vi "GUI_FINAL.vi"() -> ()   [LabVIEW 2013]
uses:
  <vilib>/userdefined/High Color/IMAQdx.ctl
  <vilib>/Instr/_visa.llb/VISA Configure Serial Port (Instr).vi
  <vilib>/vision/driver/NI_Vision_Acquisition_Software.lvlib
panel:
  out "Temperatura Alta":bool
  out "Nivel Bajo":bool
  in  "CAMARA RETRO":bool
  out "luces":u8
  out "Gasolina":u8(slide) scale=0.0..100.0
  out "Capturaretro":T1(plugin-control)
  out "Direccional  Izquierda 2":bool
  out "Direccional Derecha 2":bool
  out "FRENO":bool
  out "LUZ DELANTERA":bool
  in  "ENCENDER":bool[](array[boolean])
  in  "VISA resource name":refnum<visa-resource-name>
  in  "stop":bool
  out "Hora":string
  out "Fecha":string
  out "velocidad":u8
  out "Km recorridos":u8
  out "nivel":u8
  out "temperatura":u8
  out "Vel":dbl(knob) scale=0.0..160.0
  out "Temperatura":dbl(knob) scale=0.0..100.0
  out "error out":errorcluster
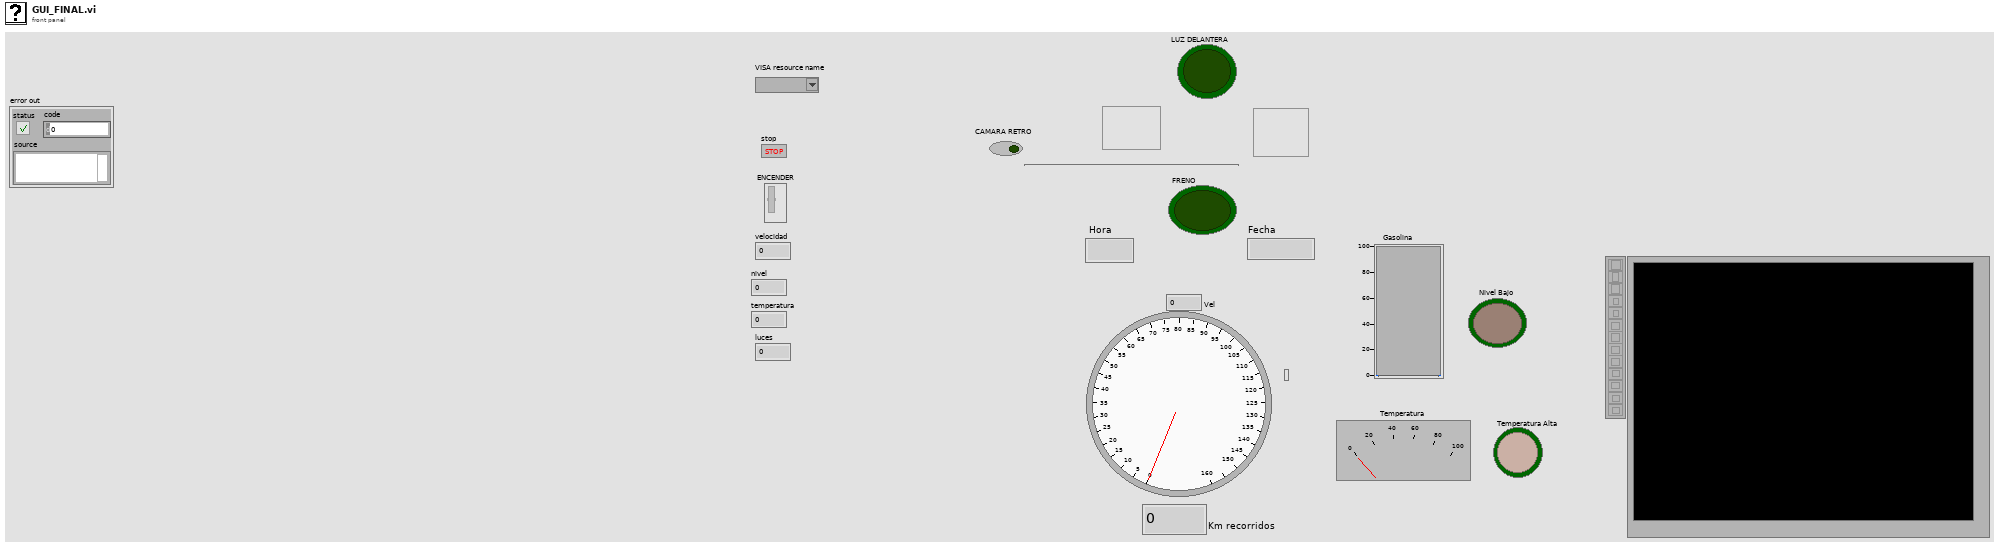
[diagram p1: front panel]
types:
  T1 = typedef "IMAQ Image.ctl" = refnum<image>
  T2 = typedef "IMAQdx.ctl" = refnum<k21>
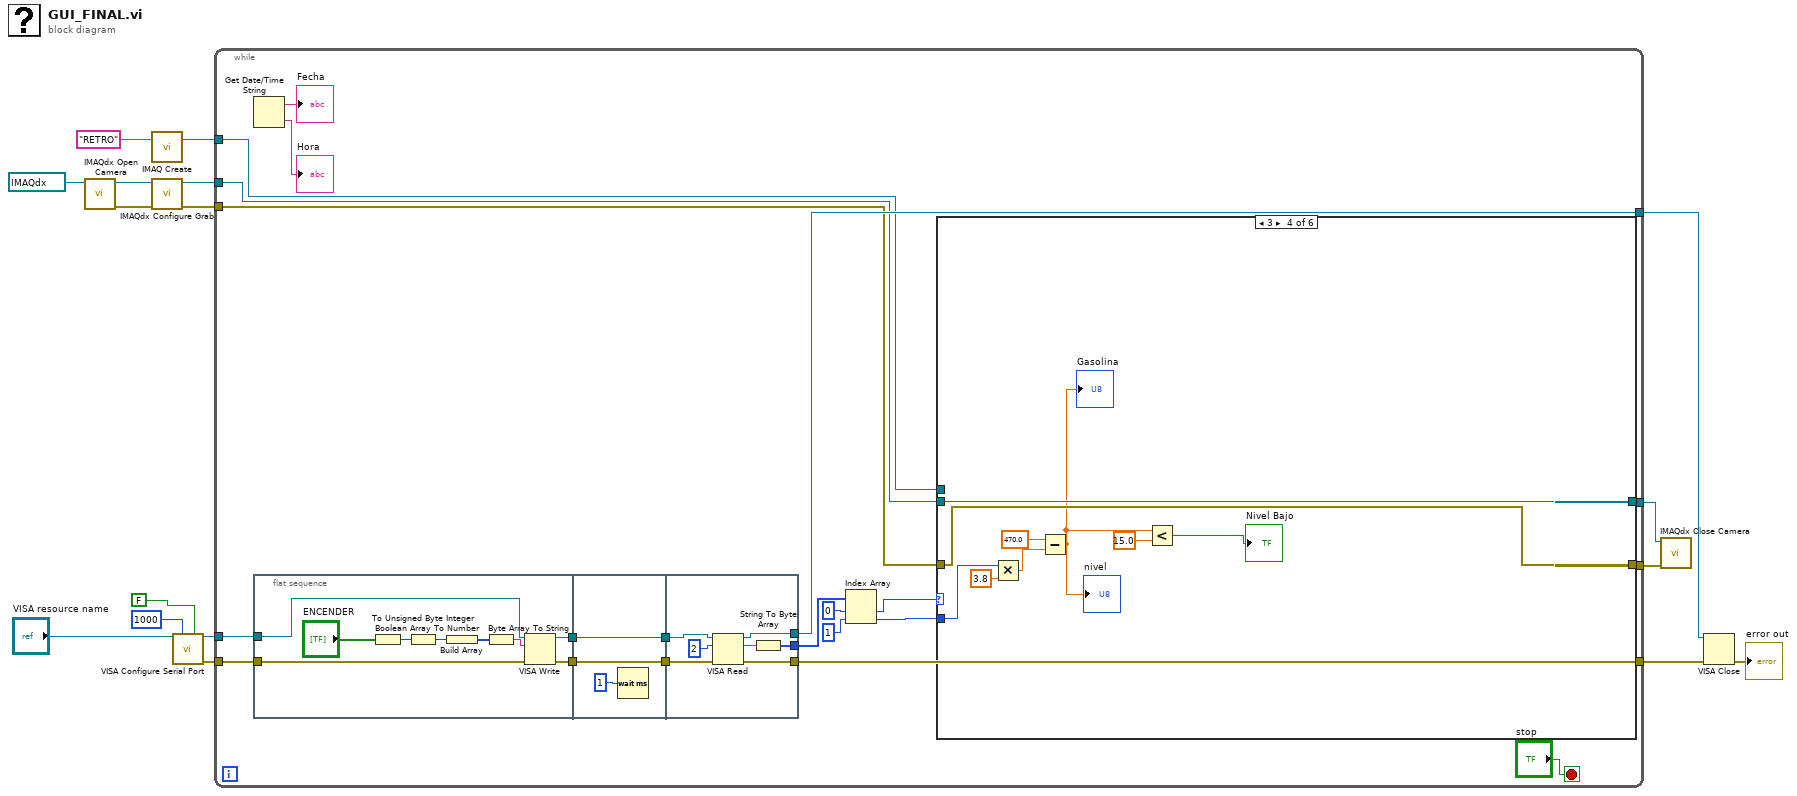
[diagram p0: block diagram]
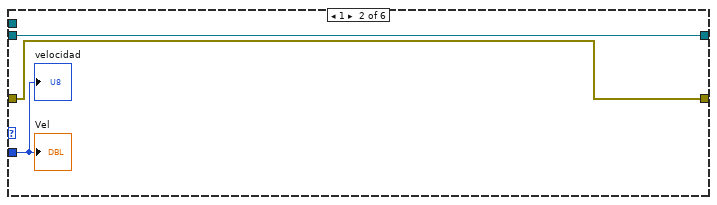
[diagram p3: hidden frame]
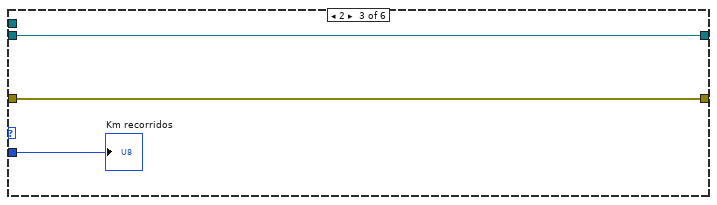
[diagram p4: hidden frame]
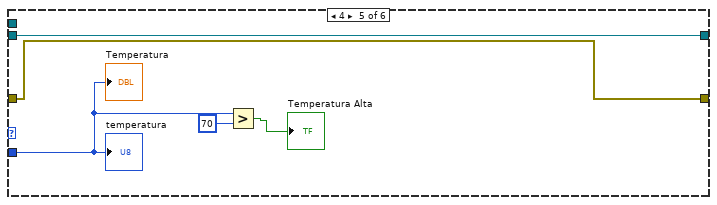
[diagram p5: hidden frame]
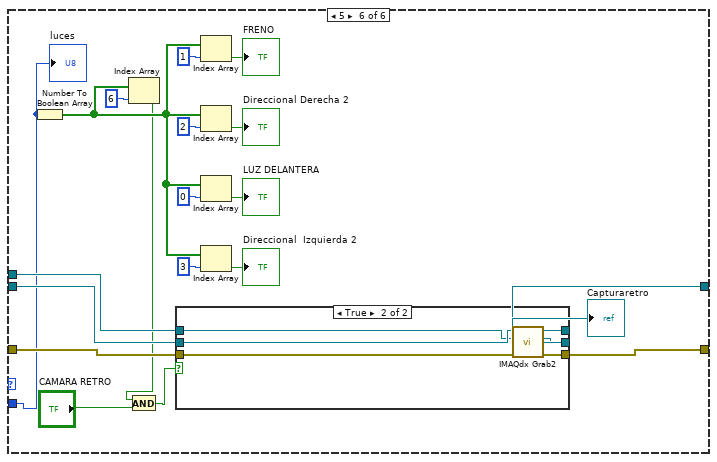
[diagram p6: hidden frame]
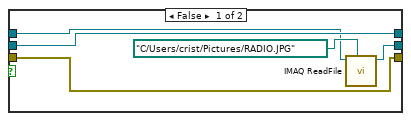
[diagram p7: hidden frame]
diagram:
  n1 = call <vilib>:"IMAQdx Open Camera.vi"("Session In"=T2 "cam5") -> ("error out"=w16:errorcluster, "Session Out"=w15:T2)  [unwired: 9 in]
  n2 = call "IMAQ Create"("Image Name"="RETRO") -> ("New Image"=w12:T1)  [unwired: 4 in, 1 out]
  n3 = call <vilib>:"IMAQdx Configure Grab.vi"("error in"=w16, "Session In"=w15) -> ("error out"=w11:errorcluster, "Session Out"=w13:T2)  [unwired: 8 in]
  n4 = call-poly "VISA Configure Serial Port"("VISA resource name"="VISA resource name", "timeout (10sec)"=u32 1000, "Enable Termination\nChar (T)"=FALSE ("Enable Termination\nChar (T)")) -> ("VISA resource name out"=w5:refnum<visa-resource-name>, "error out"=w4:errorcluster)  [unwired: 11 in]
  n5 = while {
    tunnel: w5 -> [w30]
    tunnel: w13 -> [w22]
    tunnel: w11 -> [w21]
    tunnel: w12 -> [w20]
    tunnel: [w18] -> w10
    tunnel: [w19] -> w9
    tunnel: w4 -> [w31]
    tunnel: [w29] -> w2
    tunnel: [w28] -> w1
    stop <- "stop" stop-if-true
    n6 = Get Date/Time String() -> (date string=→"Fecha":string, time string=→"Hora":string)  [unwired: 3 in]
    n7 = flat-sequence {
      tunnel: w30 -> [w47]
      tunnel: w31 -> [w46]
      tunnel: [w45] -> w35
      tunnel: [w44] -> w34
      tunnel: w35 -> [w49]
      tunnel: [w49] -> w33
      tunnel: w34 -> [w48]
      tunnel: [w48] -> w32
      tunnel: [w56] -> w28
      tunnel: [w55] -> w29
      tunnel: [w53] -> w26
      tunnel: w33 -> [w52]
      tunnel: w32 -> [w51]
      frame #0 {
        n8 = Boolean Array To Number(Boolean array="ENCENDER") -> (number=w42:u32)
        n9 = To Unsigned Byte Integer(number=w42) -> (unsigned 8bit integer=w41:u8)
        n10 = Build Array(w41) -> (w43:u8[])
        n11 = Byte Array To String(unsigned byte array=w43) -> (string=w40:string)
        n12 = VISA Write(VISA resource name=w47, write buffer=w40, error in (no error)=w46) -> (VISA resource name out=w45:refnum<visa-resource-name>, error out=w44:errorcluster)  [unwired: 1 out]
      }
      frame #1 {
        n13 = Wait (ms)(milliseconds to wait=u32 1) -> ()  [unwired: 1 out]
      }
      frame #2 {
        n14 = VISA Read(VISA resource name=w52, byte count=u32 2, error in (no error)=w51) -> (VISA resource name out=w56:refnum<visa-resource-name>, read buffer=w54:string, error out=w55:errorcluster)  [unwired: 1 out]
        n15 = String To Byte Array(string=w54) -> (unsigned byte array=w53:u8[])
      }
    }
    n16 = Index Array(array=w26, index #1=0 ("index"), index #2=1 ("index")) -> (element #1=w24:u8, element #2=w23:u8)
    n17 = case shown="3" w24 {
      tunnel: w23 -> [_ w62 w65 w72 w77 w84]
      tunnel: w22 -> [w58 w60 w63 w73 w78 w89]
      tunnel: w21 -> [w59 w61 w64 w74 w79 w88]
      tunnel: w20 -> [_ _ _ _ _ w87]
      tunnel: [w58 w60 w63 w73 w78 w86] -> w19
      tunnel: [w59 w61 w64 w74 w79 w85] -> w18
      frame 0, Default {
      }
      frame 1 {
        "velocidad" <- w62
        "Vel" <- w62
      }
      frame 2 {
        "Km recorridos" <- w65
      }
      frame 3 {
        n18 = Multiply(x=w72, y=3.8) -> (x*y=w70:dbl)
        n19 = Subtract(x=470.0, y=w70) -> (x-y=w68:dbl)
        "nivel" <- w68
        "Gasolina" <- w68
        n20 = Less?(x=w68, y=15.0) -> (x < y?=→"Nivel Bajo":bool)
      }
      frame 4 {
        n21 = Greater?(x=w77, y=u8 70) -> (0:→"Temperatura Alta":bool)
        "temperatura" <- w77
        "Temperatura" <- w77
      }
      frame 5 {
        n22 = Number To Boolean Array(number=w84) -> (Boolean array=w83:bool[])
        n23 = Index Array(array=w83, index=6) -> (element=w82:bool)
        n24 = And(x=w82, y="CAMARA RETRO") -> (x .and. y?=w80:bool)
        n25 = case shown="True" w80 {
          tunnel: [w102 w110] -> w86
          tunnel: [w100 w108] -> w85
          tunnel: [w104 w109] -> w90
          tunnel: w89 -> [w102 w107]
          tunnel: w87 -> [w101 w106]
          tunnel: w88 -> [w100 w105]
          frame False {
            n26 = call "IMAQ ReadFile"("File Path"=path "C:/Users/crist/Pictures/RADIO.JPG", "Image"=w101) -> ("Image Out"=w104:T1)  [unwired: 5 in, 4 out]
          }
          frame True {
            n27 = call <vilib>:"IMAQdx Grab2.vi"("error in"=w105, "Image In"=w106, "Session In"=w107) -> ("error out"=w108:errorcluster, "Image Out"=w109:T1, "Session Out"=w110:T2)  [unwired: 5 in, 1 out]
          }
        }
        "Capturaretro" <- w90
        n28 = Index Array(array=w83, index=1) -> (element=→"FRENO":bool)
        n29 = Index Array(array=w83, index=2) -> (element=→"Direccional Derecha 2":bool)
        n30 = Index Array(array=w83, index=0) -> (element=→"LUZ DELANTERA":bool)
        n31 = Index Array(array=w83, index=3) -> (element=→"Direccional  Izquierda 2":bool)
        "luces" <- w84
      }
    }
  }
  n32 = call <vilib>:"IMAQdx Close Camera.vi"("error in"=w10, "Session In"=w9) -> ()  [unwired: 9 in, 1 out]
  n33 = VISA Close(VISA resource name=w1, error in (no error)=w2) -> (error out=→"error out":errorcluster)
